vi "Create Channels.vi"(8 "error in (no error)":errorcluster, 11 "FunctionGenerator in":refnum<class "FunctionGenerator.lvclass">) -> (0 "error out":errorcluster, 3 "FunctionGenerator out":refnum<class "FunctionGenerator.lvclass">)   [LabVIEW 2019, in "FunctionGenerator.lvlib" / "FunctionGenerator.lvclass"]
uses:
  Library/FunctionGenerator.lvclass
  Custom Controls/WaveformSettings.ctl
  Custom Controls/WaveformMode.ctl
  Library/FunctionGenerator.lvclass/FunctionGenerator.ctl
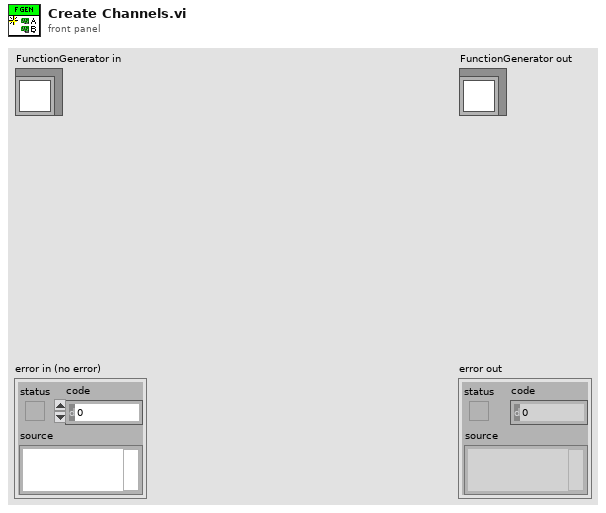
[diagram p1: front panel]
types:
  T1 = typedef "FunctionGenerator.lvlib/FunctionGenerator.lvclass/WaveformSettings.ctl" = cluster{"Frequency":dbl, "Amplitude":dbl, "Offset":dbl, "Phase":dbl, "Symmetry":dbl, "Pulse Width":dbl, "Rise Time":dbl, "Fall Time":dbl, "Mode":T2, "Termination":enum16{"50_Ohm", "High_Z"}, "Output":bool}
  T2 = typedef "FunctionGenerator.lvlib/FunctionGenerator.lvclass/WaveformMode.ctl" = enum16{"Sine", "Square", "Ramp", "Pulse", "Arbitrary", "Triangle", "Noise", "DC"}
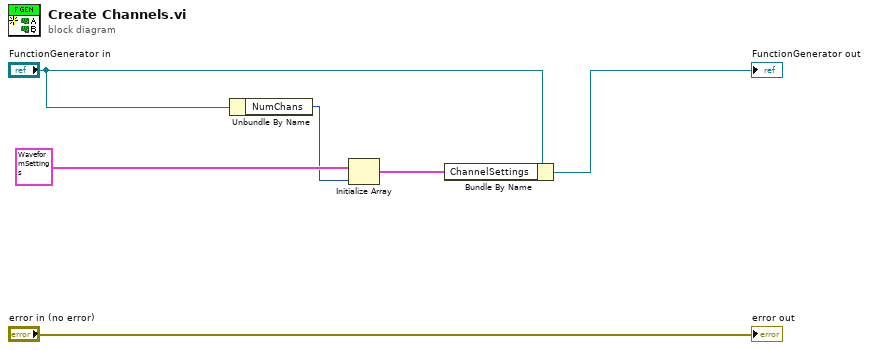
[diagram p0: block diagram]
diagram:
  n1 = Unbundle By Name("FunctionGenerator in") -> ("NumChans"=w3:i32)
  n2 = Initialize Array(T1 {"Frequency"=0.0, "Amplitude"=0.0, "Offset"=0.0, "Phase"=0.0, "Symmetry"=0.0, "Pulse Width"=0.0, "Rise Time"=0.0, "Fall Time"=0.0, "Mode"=enum."Sine", "Termination"=enum."50_Ohm", "Output"=FALSE} ("Settings"), w3) -> (w2:T1[])
  n3 = Bundle By Name(cluster="FunctionGenerator in", "ChannelSettings"=w2) -> (→"FunctionGenerator out":refnum<class "FunctionGenerator.lvclass">)
  "error out" <- "error in (no error)"
